vi "GetSetTemperatureScale.vi"(0 "VISA resource name":refnum<visa-resource-name>, 5 "get/set":T2=enum."set", 9 "Temperature scale":T1 items=["Celsius", "Fahrenheit"], 11 "error in":errorcluster) -> (4 "VISA resource name out":refnum<visa-resource-name>, 6 "Temperature scale string\n(0=Celsius; 1=Fahrenheit)":string, 8 "Temperature scale\n(0=Celsius; 1=Fahrenheit)":u8, 10 "Temperature scale text":string, 15 "error out":errorcluster)   [LabVIEW 2023, in "Thermotron 8800.lvlib"]
doc: "TMPS\nCommand name: Send or load temperature scale\nCommand type: Variable\nDescription: Allows you to read or change the temperature scale used on the 8800 display. NOTE: This command does not affect the 8800 interface commands.\nSyntax: TMPS?\nData type: Coded integer (0 = Celsius, 1 = Fahrenheit)\nQuery example: TMPS?\n8800 response: 0 (The temperature scale used on the 8800 display is Celsius.)\nOperation example: TMPS1\n8800 response: The 8800 sets the temperature scale to Fahrenheit."
uses:
  Thermotron 8800.lvlib
  Private/get set.ctl
  Private/Celcius or Fahrenheit.ctl
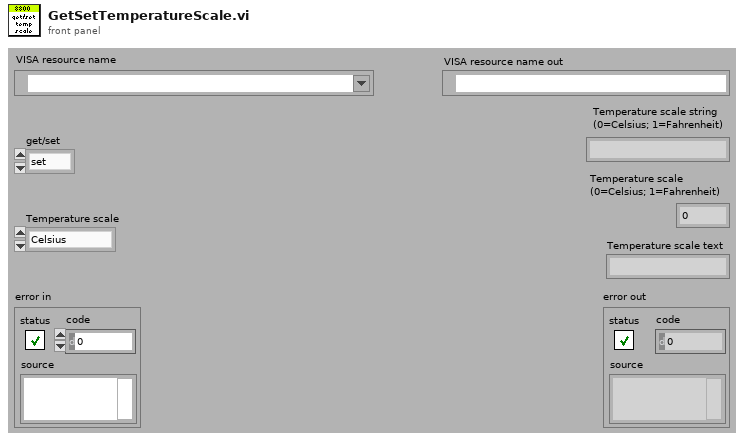
[diagram p1: front panel]
types:
  T1 = typedef "Thermotron 8800.lvlib/Celcius or Fahrenheit.ctl" = u8
  T2 = typedef "Thermotron 8800.lvlib/get set.ctl" = enum16{"get", "set"}
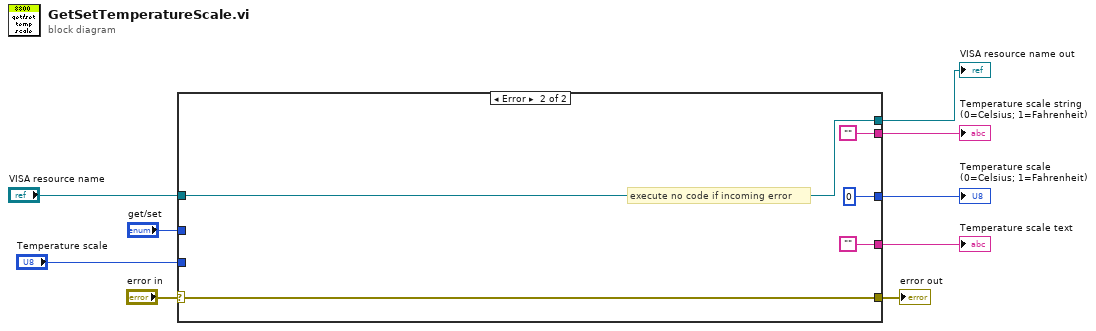
[diagram p0: block diagram]
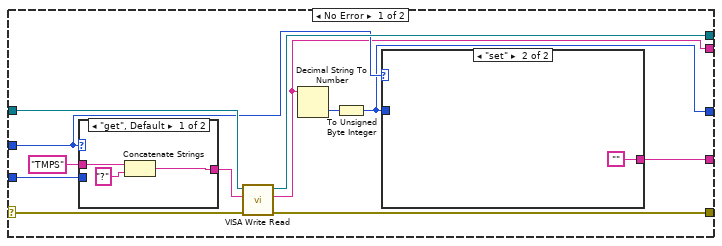
[diagram p2: hidden frame]
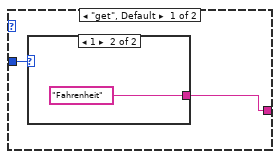
[diagram p3: hidden frame]
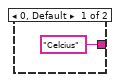
[diagram p4: hidden frame]
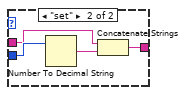
[diagram p5: hidden frame]
diagram:
  n1 = case shown="Error" "error in" {
    selector: "error in" -> [w17 w38]
    tunnel: [w20 w38] -> w9
    tunnel: [w19 w37] -> w8
    tunnel: "VISA resource name" -> [w18 w37]
    tunnel: "get/set" -> [w14 _]
    tunnel: [w12 ""] -> w5
    tunnel: "Temperature scale" -> [w16 _]
    tunnel: [w10 u8 0] -> w2
    tunnel: [w13 ""] -> w1
    frame No Error {
      n2 = case shown="\"get\", Default" w14 {
        tunnel: [w29 w30] -> w21
        tunnel: w16 -> [_ w33]
        tunnel: "TMPS" ("8800 Command") -> [w27 w31]
        frame "get", Default {
          n3 = Concatenate Strings(w27, "?" ("8800 Command")) -> (w29:string)
        }
        frame "set" {
          n4 = Number To Decimal String(number=w33) -> (decimal integer string=w32:string)  [unwired: 1 in]
          n5 = Concatenate Strings(w31, w32) -> (w30:string)
        }
      }
      n6 = call "VISA Write Read.vi"("error in (no error)"=w17, "8800 Command"=w21, "VISA Refnum in"=w18) -> ("error out"=w20:errorcluster, "read buffer"=w12:string, "VISA Refnum out"=w19:refnum<visa-resource-name>)  [unwired: 6 in]
      n7 = Decimal String To Number(string=w12) -> (number=w11:i32)  [unwired: 2 in, 1 out]
      n8 = To Unsigned Byte Integer(number=w11) -> (unsigned 8bit integer=w10:u8)
      n9 = case shown="\"set\"" w14 {
        tunnel: [w23 ""] -> w13
        tunnel: w10 -> [w22 _]
        frame "get", Default {
          n10 = case shown="1" w22 {
            tunnel: ["Celcius" "Fahrenheit"] -> w23
            frame 0, Default {
            }
            frame 1 {
            }
          }
        }
        frame "set" {
        }
      }
    }
    frame Error {
      # "execute no code if incoming error"
    }
  }
  "VISA resource name out" <- w8
  "error out" <- w9
  "Temperature scale string\n(0=Celsius; 1=Fahrenheit)" <- w5
  "Temperature scale\n(0=Celsius; 1=Fahrenheit)" <- w2
  "Temperature scale text" <- w1
